vi "Create Query Message.vi"(11 "query":T1 {"header"."opcode" items=["Query"=0, "IQuery"=1, "Status"=2, "Notify"=4, "Update"=5, "DSO"=6]; "questions"."class" items=["IN"=1, "CH"=3, "HS"=4, "NONE"=254, "*"=255]; "questions"."type" items=["A"=1, "NS"=2, "MD"=3, "MF"=4, "CNAME"=5, "SOA"=6, "MB"=7, "MG"=8, "MR"=9, "NULL"=10, "WKS"=11, "PTR"=12, "HINFO"=13, "MINFO"=14, "MX"=15, "TXT"=16, "RP"=17, "AFSDB"=18, "X25"=19, "ISDN"=20, "RT"=21, "NSAP"=22, "NSAP-PTR"=23, "SIG"=24, "KEY"=25, "PX"=26, "GPOS"=27, "AAAA"=28, "LOC"=29, "NXT"=30, "EID"=31, "NIMLOC"=32, "SRV"=33, "ATMA"=34, "NAPTR"=35, "KX"=36, "CERT"=37, "A6"=38, "DNAME"=39, "SINK"=40, "OPT"=41, "APL"=42, "DS"=43, "SSHFP"=44, "IPSECKEY"=45, "RRSIG"=46, "NSEC"=47, "DNSKEY"=48, "DHCID"=49, "NSEC3"=50, "NSEC3PARAM"=51, "TLSA"=52, "SMIMEA"=53, "HIP"=55, "NINFO"=56, "RKEY"=57, "TALINK"=58, "CDS"=59, "CDNSKEY"=60, "OPENPGPKEY"=61, "CSYNC"=62, "ZONEMD"=63, "SVCB"=64, "HTTPS"=65, "SPF"=99, "UINFO"=100, "UID"=101, "GID"=102, "UNSPEC"=103, "NID"=104, "L32"=105, "L64"=106, "LP"=107, "EUI48"=108, "EUI64"=109, "TKEY"=249, "TSIG"=250, "IXFR"=251, "AXFR"=252, "MAILB"=253, "MAILA"=254, "*"=255, "URI"=256, "CAA"=257, "AVC"=258, "DOA"=259, "AMTRELAY"=260, "TA"=32768, "DLV"=32769]}) -> (3 "message":string)   [LabVIEW 2015, in "PL DNS Client.lvlib"]
doc: "Creates DNS query <b>message</b>."
uses:
  PL DNS Client.lvlib
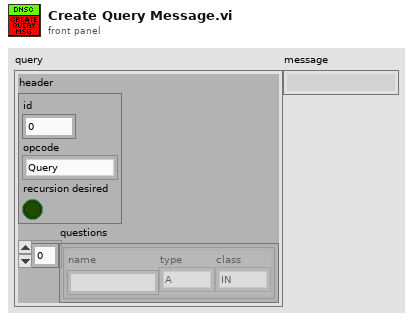
[diagram p1: front panel]
types:
  T1 = cluster{"header":cluster{"id":u16, "opcode":u8, "recursion desired":bool}, "questions":cluster{"name":string, "type":u16, "class":u16}[]}
  T2 = cluster{"name":string, "type":u16, "class":u16}[]
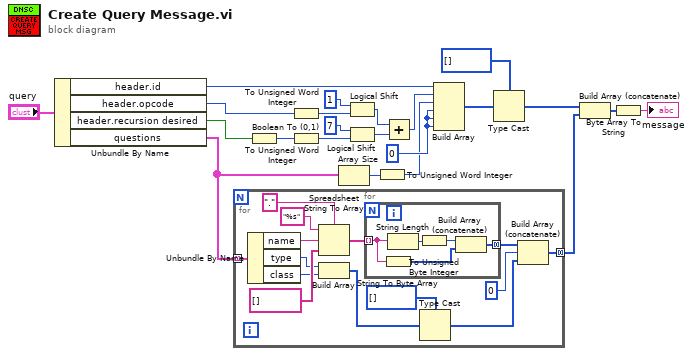
[diagram p0: block diagram]
diagram:
  w20 = u16 0
  n1 = Unbundle By Name("query") -> ("header.id"=w5:u16, "header.opcode"=w4:u8, "header.recursion desired"=w3:bool, "questions"=w2:T2)
  n2 = for {
    tunnel: w2 -> [w30] mode=indexing
    tunnel: [w23] -> w9 mode=concatenating
    n3 = Unbundle By Name(w30) -> ("name"=w29:string, "type"=w28:u16, "class"=w27:u16)
    n4 = Spreadsheet String To Array(delimiter (Tab)=".", format string="%s", spreadsheet string=w29, array type (2D Dbl)=string[] []) -> (array=w33:string[])
    n5 = Build Array(w28, w27) -> (w25:u16[])
    n6 = for {
      tunnel: w33 -> [w41] mode=indexing
      tunnel: [w37] -> w32 mode=concatenating
      n7 = String To Byte Array(string=w41) -> (unsigned byte array=w38:u8[])
      n8 = String Length(string=w41) -> (length=w40:i32)
      n9 = To Unsigned Byte Integer(number=w40) -> (unsigned 8bit integer=w39:u8)
      n10 = Build Array (concatenate)(w39, w38) -> (w37:u8[])
    }
    n11 = Type Cast(type=u8[] [], x=w25) -> (*(type *) &x=w24:u8[])
    n12 = Build Array (concatenate)(w32, u8 0 ("unsigned 8bit integer"), w24) -> (w23:u8[])
  }
  n13 = Boolean To (0,1)(Boolean=w3) -> (0, 1=w18:i16)
  n14 = To Unsigned Word Integer(number=w4) -> (unsigned 16bit integer=w10:u16)
  n15 = To Unsigned Word Integer(number=w18) -> (unsigned 16bit integer=w16:u16)
  n16 = Array Size(array=w2) -> (size(s)=w12:i32)
  n17 = Logical Shift(y=i16 1, x=w10) -> (x << y=w15:u16)
  n18 = Logical Shift(y=i16 7, x=w16) -> (x << y=w14:u16)
  n19 = To Unsigned Word Integer(number=w12) -> (unsigned 16bit integer=w11:u16)
  n20 = Add(x=w15, y=w14) -> (x+y=w13:u16)
  n21 = Build Array(w5, w13, w11, w20, w20, w20) -> (w7:u16[])
  n22 = Type Cast(type=u8[] [] ("array"), x=w7) -> (*(type *) &x=w22:u8[])
  n23 = Build Array (concatenate)(w22, w9) -> (w8:u8[])
  n24 = Byte Array To String(unsigned byte array=w8) -> (string=→"message":string)
